vi "SDKSID4_Stop Live Mode.vi"(4 "error in (no error)":errorcluster, 7 "SDKSID4 session In":T1) -> (0 "error out":errorcluster, 3 "SDKSID4 session Out":T1)   [LabVIEW 2013]
doc: "This VI stops a camera session previously opened with Start Live Mode. Use this VI when a measurement session is finished in order to make the camera return to the idle mode."
uses:
  Refnum SDKSID4 session.ctl
  SID4_SDK.dll
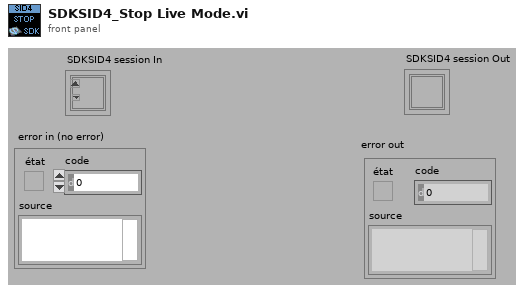
[diagram p1: front panel]
types:
  T1 = typedef "Refnum SDKSID4 session.ctl" = refnum<k1>
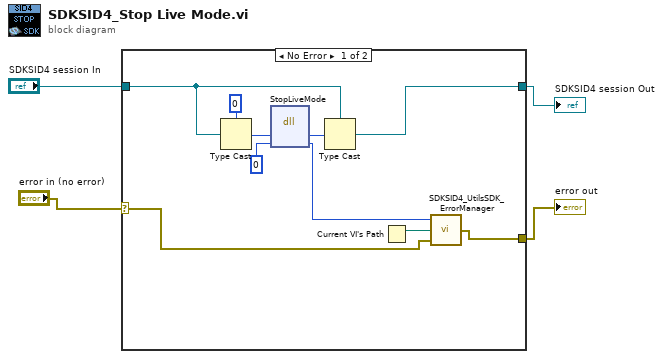
[diagram p0: block diagram]
diagram:
  n1 = case shown="No Error" "error in (no error)" {
    selector: "error in (no error)" -> [w5 w16]
    tunnel: [w6 w16] -> w1
    tunnel: "SDKSID4 session In" -> [w9 w15]
    tunnel: [w10 w15] -> w2
    frame No Error {
      n2 = Type Cast(type=u32 0, x=w9) -> (*(type *) &x=w14:u32)
      n3 = dll-call lib="C:/Program Files/SID4_SDK/DLL SDK/BIN/SID4_SDK.dll" fn="StopLiveMode"("SessionID"=w14, "Error"=0) -> ("SessionID"=w11:u32, "Error"=w7:i32)  [unwired: 4 in, 2 out]
      n4 = Type Cast(type=w9, x=w11) -> (*(type *) &x=w10:T1)
      n5 = Current VI's Path() -> (path=w8:path)
      n6 = call "SDKSID4_UtilsSDK_ErrorManager.vi"("error IN"=w5, "VI PathFile"=w8, "ErrorCode"=w7) -> ("error OUT"=w6:errorcluster)
    }
    frame Error {
    }
  }
  "SDKSID4 session Out" <- w2
  "error out" <- w1
